vi "Threshold 1D Array (xN).vi"(8 "start index (0)":dbl, 9 "Search Values":dbl[](array[numeric]), 11 "X":dbl[](array[numeric])) -> (3 "Interpolated Indices":dbl[](array[numeric]))   [LabVIEW 2021, in "Arrays.lvlib"]
uses:
  Arrays.lvlib
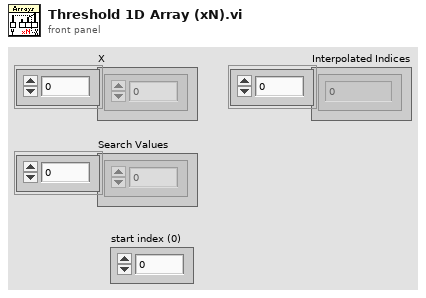
[diagram p1: front panel]
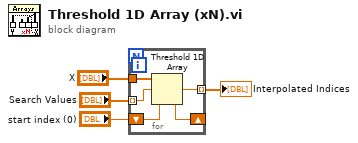
[diagram p0: block diagram]
diagram:
  n1 = for {
    tunnel: "Search Values" -> [w8] mode=indexing
    tunnel: "X" -> [w7]
    tunnel: [w5] -> w4 mode=indexing
    shift-right: [w5] -> _
    shift-left: "start index (0)" -> [w6]
    n2 = Threshold 1D Array(1:w6, 2:w8, 3:w7) -> (0:w5:dbl)
  }
  "Interpolated Indices" <- w4
